vi "FPGA cRIOMain_v3.vi"() -> ()   [LabVIEW 2019]
doc: "Main FPGA VI\nUse the bitfile generated by this VI in the real-time code.\n\nFlip the channels for input and output"
uses:
  <vilib>/eio/EIONode/EIONode.xnode
  <vilib>/rvi/DataTransferAndStorage/Container/XNode/niFpgaContainer.xnode
  <vilib>/rvi/eio/common/nirviEmuTemplateMethod_errors.vi
  <vilib>/rvi/FIFO/Fifo_Resource/nirvififoEmulationRead.vi
  <vilib>/rvi/FIFO/Fifo_Resource/nirvififoEmulationWrite.vi
  <vilib>/rvi/FXPMathLib/FxpMul/XNode/nifxpmath_Multiplier.xnode
  <vilib>/rvi/Analysis/measure/butterworth/XNode/niFpgaButterworthFilter.xnode
  FPGA functions/FPGA functions.lvlib
  <vilib>/rvi/FXPMathLib/sim/FxpSim.dll
  TypeDefs/AO mode TabCtrl.ctl
  TypeDefs/SamplingModeEnum.ctl
  TypeDefs/AI_channelEnum.ctl
panel:
  in  "Select Channel":T1
  out "Unable to\nrun at desired\nSample Time?":bool
  out "Processing Loop time [ticks]":u32
  out "FPGA AI DMA\nOverflow?":bool
  in  "Scaled Butterworth Coeffs":i32[](array[numeric])=[-1036986264, 2110353124, 93741, -1058362983, 2131726043, 94691]
  in  "Sampling Mode":T2
  in  "AO mode":T3
  in  "AO Out [V]":fxp<+/-,18,5> format="%#.6g"
  in  "AO enable?":bool
  out "AI In [V]":fxp<+/-,25,5> format="%#.6g"
  out "FPGA AO DMA\nOverflow?":bool
  out "Int. Output":fxp<+/-,20,5> format="%.17g"
  out "Raw Int. Input":fxp<+/-,24,5> format="%.21g"
  in  "Sample Time [ticks]":u32=120
  out "AO Loop time [ticks]":u32
  out "AI Loop time [ticks]":u32
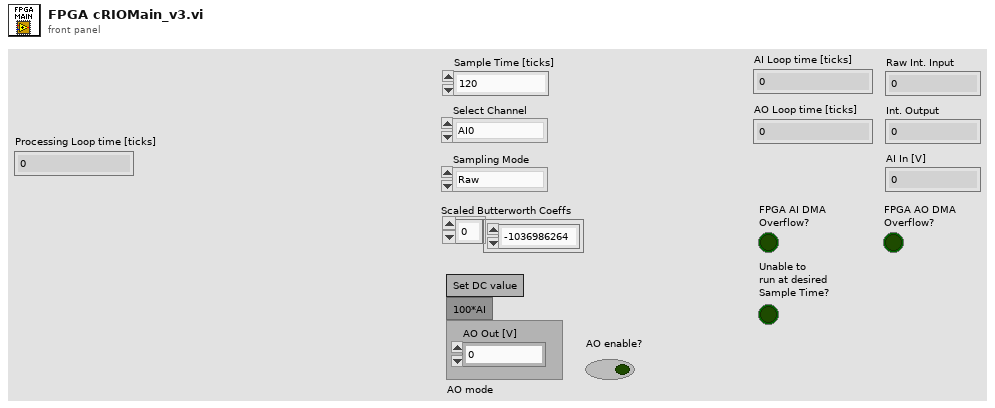
[diagram p1: front panel]
types:
  T1 = typedef "AI_channelEnum.ctl" = enum16{"AI0", "AI1", "AI2", "AI3"}
  T2 = typedef "SamplingModeEnum.ctl" = enum16{"Raw", "4pt MA (AI)", "LPF (Proc.)", "4pt MA (AI) + LPF (Proc.)", "4pt MA + LPF (Proc.)"}
  T3 = typedef "AO mode TabCtrl.ctl" = enum32{"Set DC value", "100*AI"}
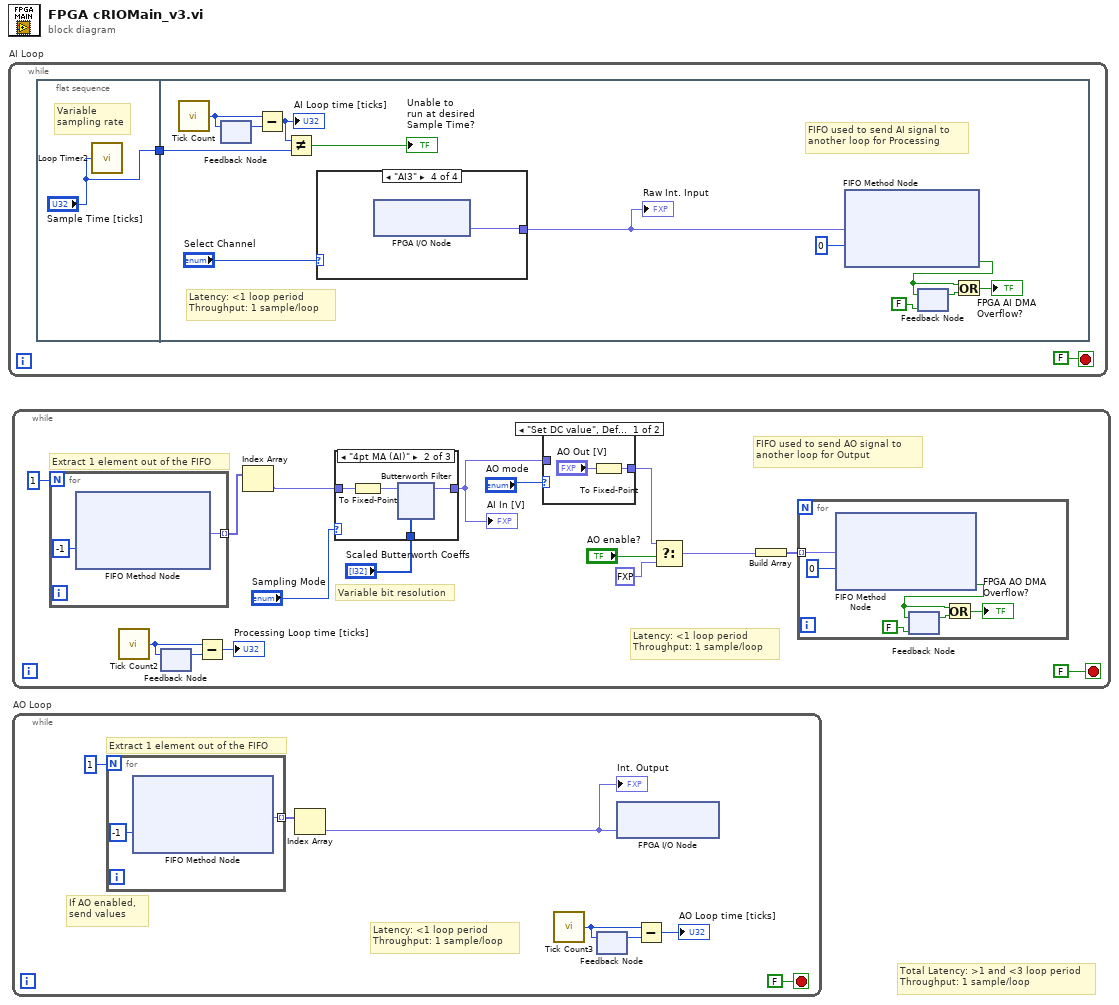
[diagram p0: block diagram]
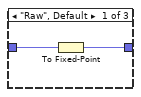
[diagram p2: hidden frame]
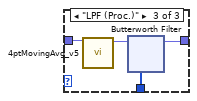
[diagram p3: hidden frame]
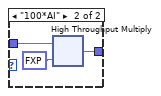
[diagram p4: hidden frame]
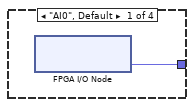
[diagram p5: hidden frame]
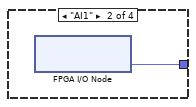
[diagram p6: hidden frame]
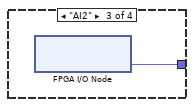
[diagram p7: hidden frame]
diagram:
  # "Total Latency: >1 and <3 loop period\nThroughput: 1 sample/loop"
  n1 = while "AI Loop" {
    stop <- FALSE stop-if-true
    n2 = flat-sequence {
      tunnel: ["Sample Time [ticks]"] -> w1
      tunnel: w1 -> [w12]
      frame #0 {
        # "Variable\nsampling rate"
        n3 = call "Loop Timer2"("Count(Ticks)"="Sample Time [ticks]") -> ()  [unwired: 1 out]
      }
      frame #1 {
        # "FIFO used to send AI signal to \nanother loop for Processing"
        # "Latency: <1 loop period\nThroughput: 1 sample/loop"
        n4 = call "Tick Count"() -> ("Tick Count(Ticks)"=w15:u32)
        n5 = feedback #1() -> (w14:u32)  [unwired: 1 in]
        n6 = feedback-in #1(w15) -> ()
        n7 = Subtract(x=w15, y=w14) -> (x-y=w13:u32)
        "AI Loop time [ticks]" <- w13
        n8 = Not Equal?(x=w13, y=w12) -> (x != y?=→"Unable to\nrun at desired\nSample Time?":bool)
        n9 = case shown="\"AI3\"" "Select Channel" {
          tunnel: [w16 w17 w18 w19] -> w4
          frame "AI0", Default {
            n10 = xnode "FPGA I/O Node"() -> ("Mod4/AI0"=w16:fxp<+/-,24,5>)  [unwired: 1 in, 1 out]
          }
          frame "AI1" {
            n11 = xnode "FPGA I/O Node"() -> ("Mod4/AI1"=w17:fxp<+/-,24,5>)  [unwired: 1 in, 1 out]
          }
          frame "AI2" {
            n12 = xnode "FPGA I/O Node"() -> ("Mod4/AI2"=w18:fxp<+/-,24,5>)  [unwired: 1 in, 1 out]
          }
          frame "AI3" {
            n13 = xnode "FPGA I/O Node"() -> ("Mod4/AI3"=w19:fxp<+/-,24,5>)  [unwired: 1 in, 1 out]
          }
        }
        "Raw Int. Input" <- w4
        n14 = xnode ("FIFO Method Node")("Element"=w4, "Timeout"=0) -> ("Timed Out?"=w5:bool)  [unwired: 1 in, 1 out]
        n15 = feedback #2(FALSE ("Timed Out?")) -> (w8:bool)
        n16 = feedback-in #2(w5) -> ()
        n17 = Or(x=w5, y=w8) -> (x .or. y?=→"FPGA AI DMA\nOverflow?":bool)
      }
    }
  }
  n18 = while {
    stop <- FALSE stop-if-true
    # "Extract 1 element out of the FIFO"
    # "Variable bit resolution"
    # "Latency: <1 loop period\nThroughput: 1 sample/loop"
    # "FIFO used to send AO signal to \nanother loop for Output"
    n19 = for {
      N: 1 -> [_]
      tunnel: [w37] -> w25 mode=indexing
      n20 = xnode ("FIFO Method Node")("Timeout"=-1) -> ("Element"=w37:fxp<+/-,24,5>)  [unwired: 1 in, 2 out]
    }
    n21 = call "Tick Count2"() -> ("Tick Count(Ticks)"=w24:u32)
    n22 = feedback #3() -> (w23:u32)  [unwired: 1 in]
    n23 = feedback-in #3(w24) -> ()
    n24 = Subtract(x=w24, y=w23) -> (x-y=→"Processing Loop time [ticks]":u32)
    n25 = Index Array(array=w25) -> (element=w26:fxp<+/-,24,5>)  [unwired: 1 in]
    n26 = case shown="\"4pt MA (AI)\"" "Sampling Mode" {
      tunnel: w26 -> [w38 w41 w53]
      tunnel: "Scaled Butterworth Coeffs" -> [_ w43 w55]
      tunnel: [w39 w42 w54] -> w28
      frame "Raw", Default {
        n27 = To Fixed-Point(number=w38) -> (fixed-point=w39:fxp<+/-,25,5>)  [unwired: 1 in]
      }
      frame "4pt MA (AI)" {
        n28 = To Fixed-Point(number=w41) -> (fixed-point=w40:fxp<+/-,25,5>)  [unwired: 1 in]
        n29 = xnode "Butterworth Filter"("input data"=w40, "scaled coefficients"=w43) -> ("output data"=w42:fxp<+/-,25,5>)  [unwired: 1 in]
      }
      frame "LPF (Proc.)" {
        n30 = call "4ptMovingAvg_v5.vi"("Raw input"=w53) -> ("Avg. output"=w52:fxp<+/-,25,5>)  [unwired: 10 in]
        n31 = xnode "Butterworth Filter"("input data"=w52, "scaled coefficients"=w55) -> ("output data"=w54:fxp<+/-,25,5>)  [unwired: 1 in]
      }
    }
    "AI In [V]" <- w28
    n32 = case shown="\"Set DC value\", Default" "AO mode" {
      tunnel: [w65 w66] -> w32
      tunnel: w28 -> [_ w68]
      frame "Set DC value", Default {
        n33 = To Fixed-Point(number="AO Out [V]") -> (fixed-point=w65:fxp<+/-,20,5>)  [unwired: 1 in]
      }
      frame "100*AI" {
        n34 = xnode ("High Throughput Multiply")("x"=w68, "y"=fxp<+,5,7> 100.0) -> ("x*y"=w66:fxp<+/-,20,5>)
      }
    }
    n35 = Select(t=w32, s="AO enable?", f=fxp<+/-,20,5> 0.0) -> (s? t:f=w20:fxp<+/-,20,5>)
    n36 = Build Array(w20) -> (w33:fxp<+/-,20,5>[])
    n37 = for {
      tunnel: w33 -> [w69] mode=indexing
      n38 = xnode ("FIFO Method Node")("Element"=w69, "Timeout"=0) -> ("Timed Out?"=w70:bool)  [unwired: 1 in, 1 out]
      n39 = feedback-in #4(w70) -> ()
      n40 = feedback #4(FALSE ("Timed Out?")) -> (w73:bool)
      n41 = Or(x=w70, y=w73) -> (x .or. y?=→"FPGA AO DMA\nOverflow?":bool)
    }
  }
  n42 = while "AO Loop" {
    stop <- FALSE stop-if-true
    # "Latency: <1 loop period\nThroughput: 1 sample/loop"
    # "If AO enabled, \nsend values"
    # "Extract 1 element out of the FIFO"
    n43 = for {
      N: 1 -> [_]
      tunnel: [w83] -> w77 mode=indexing
      n44 = xnode ("FIFO Method Node")("Timeout"=-1) -> ("Element"=w83:fxp<+/-,20,5>)  [unwired: 1 in, 2 out]
    }
    n45 = Index Array(array=w77) -> (element=w75:fxp<+/-,20,5>)  [unwired: 1 in]
    "Int. Output" <- w75
    n46 = call "Tick Count3"() -> ("Tick Count(Ticks)"=w80:u32)
    n47 = feedback #5() -> (w79:u32)  [unwired: 1 in]
    n48 = feedback-in #5(w80) -> ()
    n49 = xnode "FPGA I/O Node"("Mod3/AO1"=w75) -> ()  [unwired: 1 in, 1 out]
    n50 = Subtract(x=w80, y=w79) -> (x-y=→"AO Loop time [ticks]":u32)
  }
